vi "Get Channel Unit.vi"(9 "Position_RVDT_Properties":T1 {"Sensitivity Units" items=["mVolts/Volt/Degree"=12507, "mVolts/Volt/Radian"=12508]; "Units" items=["Degrees"=10146, "Radians"=10273, "From Custom Scale"=10065]; "Excitation Sense" items=["Local"=16095, "Remote"=16096]; "Excitation Source" items=["Internal"=10200, "External"=10167, "None"=10230]; "Excitation Wire Mode" items=["4-Wire"=4, "5-Wire"=5, "6-Wire"=6]}, 10 "Position_LVDT_Properties":T2 {"Excitation Sense" items=["Local"=16095, "Remote"=16096]; "Excitation Source" items=["Internal"=10200, "External"=10167, "None"=10230]; "Excitation Wire Mode" items=["4-Wire"=4, "5-Wire"=5, "6-Wire"=6]; "Units" items=["Meters"=10219, "Inches"=10379, "From Custom Scale"=10065]; "Sensitivity Units" items=["mVolts/Volt/mMeter"=12506, "mVolts/Volt/0.001 Inch"=12505]}, 11 "Measurement Type":i32(ring) items=["Position LVDT", "Position RVDT"]) -> (2 "Sensitivity Unit":string, 3 "Channel Unit":string)   [LabVIEW 2020, in "NI PXIe-4340 System Explorer.lvlib"]
uses:
  NI PXIe-4340 System Explorer.lvlib
  Shared/Position_LVDT_Properties.ctl
  Shared/Position_RVDT_Properties.ctl
  Shared/NI PXIe-4340 Shared.lvlib
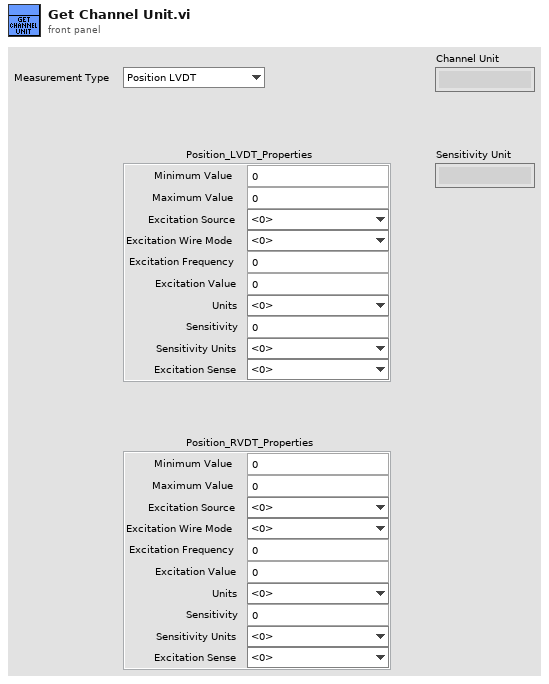
[diagram p1: front panel]
types:
  T1 = typedef "NI PXIe-4340 Shared.lvlib/Position_RVDT_Properties.ctl" = cluster{"Minimum Value":dbl, "Maximum Value":dbl, "Excitation Source":i32, "Excitation Wire Mode":i32, "Excitation Frequency":dbl, "Excitation Value":dbl, "Units":i32, "Sensitivity":dbl, "Sensitivity Units":i32, "Excitation Sense":i32}
  T2 = typedef "NI PXIe-4340 Shared.lvlib/Position_LVDT_Properties.ctl" = cluster{"Minimum Value":dbl, "Maximum Value":dbl, "Excitation Source":i32, "Excitation Wire Mode":i32, "Excitation Frequency":dbl, "Excitation Value":dbl, "Units":i32, "Sensitivity":dbl, "Sensitivity Units":i32, "Excitation Sense":i32}
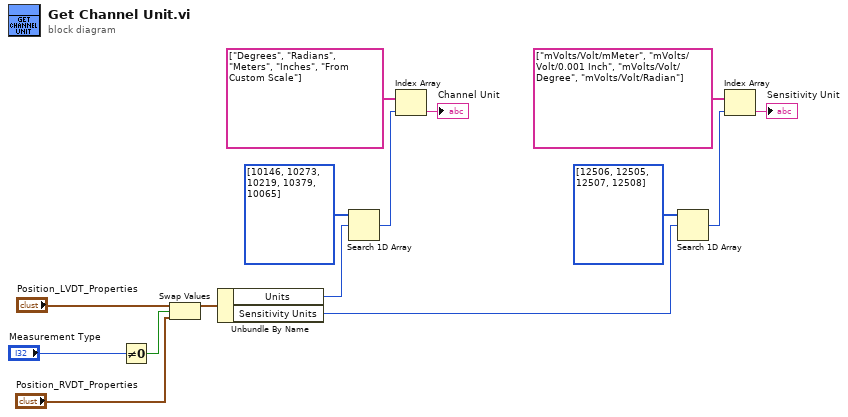
[diagram p0: block diagram]
diagram:
  n1 = Not Equal To 0?(x="Measurement Type") -> (x != 0?=w10:bool)
  n2 = Swap Values(12:"Position_LVDT_Properties", 13:w10, 14:"Position_RVDT_Properties") -> (1:w9:T2)  [unwired: 1 out]
  n3 = Unbundle By Name(w9) -> ("Units"=w12:i32, "Sensitivity Units"=w1:i32)
  n4 = Search 1D Array(1D array=i32[] [10146, 10273, 10219, 10379, 10065], element=w12) -> (index of element=w13:i32)  [unwired: 1 in]
  n5 = Index Array(array=string[] ["Degrees", "Radians", "Meters", "Inches", "From Custom Scale"], index=w13) -> (element=→"Channel Unit":string)
  n6 = Search 1D Array(1D array=i32[] [12506, 12505, 12507, 12508], element=w1) -> (index of element=w4:i32)  [unwired: 1 in]
  n7 = Index Array(array=string[] ["mVolts/Volt/mMeter", "mVolts/Volt/0.001 Inch", "mVolts/Volt/Degree", "mVolts/Volt/Radian"], index=w4) -> (element=→"Sensitivity Unit":string)
